vi "Turret_Execute.vi"() -> ()   [LabVIEW 2019]
uses:
  Globals/Turret_Globals.vi
  <vilib>/Rock Robotics/WPI/ThirdParty/REV Robotics/SPARK MAX/Typedef/Spark MAX Control Type.ctl
panel:
  out "Turret_Spin_Speed":dbl
  in  "turret_spin_encoder":dbl
  in  "t_x":dbl
  in  "Kp Aim":dbl=0.08
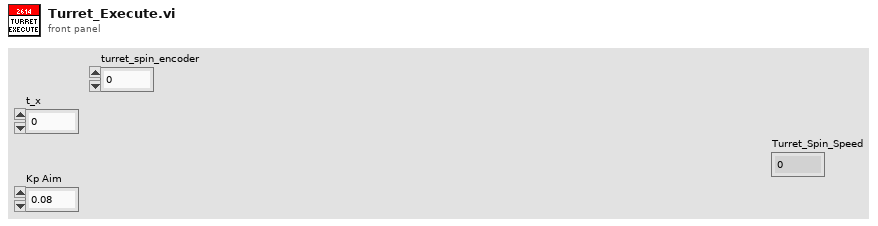
[diagram p1: front panel]
types:
  T1 = typedef "WPI_MotorControlDeviceRef.ctl" = cluster{"DeviceStatus":errorcluster, "Type":T2, "PWM":cluster{"PWM Channel":T3, "DeadBand":T4}, "CAN":cluster{"Device Number":u8, "SetOutput VI Ref":variant, "GetOutput VI Ref":variant, "Enable VI Ref":variant, "Disable VI Ref":variant, "Data":variant}, "Invert":bool, "DIO PWM":cluster{"PWM \"Enable\" Channel":T3, "DIOChannel":T5, "PWM Rate":dbl}}
  T2 = typedef "WPI_MotorControlType.ctl" = enum16{"PWM", "CAN", "DIO PWM"}
  T3 = typedef "FPGA_DIOPWMChannel.ctl" = enum8{"PWM 0", "PWM 1", "PWM 2", "PWM 3", "PWM 4", "PWM 5", "PWM 6", "PWM 7", "PWM 8", "PWM 9", "PWM MXP 0", "PWM MXP 1", "PWM MXP 2", "PWM MXP 3", "PWM MXP 4", "PWM MXP 5", "PWM MXP 6", "PWM MXP 7", "PWM MXP 8", "PWM MXP 9", "Invalid"}
  T4 = typedef "WPI_PWMDeadband.ctl" = cluster{"Name":string, "maxPositivePwm":i32, "minPositivePwm":i32, "centerPwm":i32, "maxNegativePwm":i32, "minNegativePwm":i32, "angularRange":u16}
  T5 = typedef "FPGA_DIOChannel.ctl" = enum8{"DIO 0", "DIO 1", "DIO 2", "DIO 3", "DIO 4", "DIO 5", "DIO 6", "DIO 7", "DIO 8", "DIO 9", "DIO MXP 0", "DIO MXP 1", "DIO MXP 2", "DIO MXP 3", "DIO MXP 4", "DIO MXP 5", "DIO MXP 6", "DIO MXP 7", "DIO MXP 8", "DIO MXP 9", "DIO MXP 10", "DIO MXP 11", "DIO MXP 12", "DIO MXP 13", "DIO MXP 14", "DIO MXP 15", "SPI Port CS1", "SPI Port CS2", "SPI Port CS3", "SPI Port MISO", "SPI Port MOSI", "Invalid"}
  T6 = typedef "Spark MAX Control Type.ctl" = enum16{"Percent VBus", "Voltage", "Velocity", "Position", "Smart Motion", "Current", "Smart Velocity"}
  T7 = typedef "Turret_Cluster.ctl" = cluster{"Auto-Target?":bool, "Control_State":T8, "Turret_Spin_Speed":dbl, "Turret_Spin_Speed_Control?":bool}
  T8 = typedef "Turret_States.ctl" = enum16{"Manual_Percent_Voltage", "Manual_Speed_Control", "Auto-Target"}
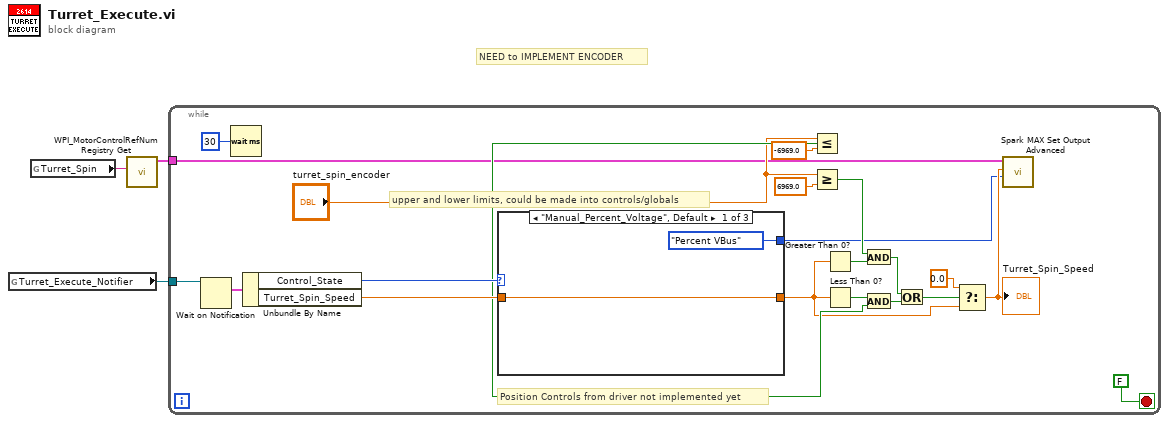
[diagram p0: block diagram]
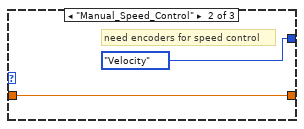
[diagram p2: hidden frame]
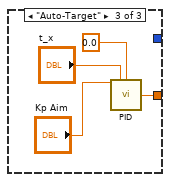
[diagram p3: hidden frame]
diagram:
  # "NEED to IMPLEMENT ENCODER"
  n1 = global read "Turret_Globals.vi" "Turret_Execute_Notifier"() -> (w3:refnum<notifier>)
  n2 = global read "Turret_Globals.vi" "Turret_Spin"() -> (w2:string)
  n3 = call <vilib>:"WPI_MotorControlRefNum Registry Get.vi"("refnum name"=w2) -> ("MotorControlDevRef"=w1:T1)  [unwired: 9 in, 1 out]
  n4 = while {
    tunnel: w3 -> [w23]
    tunnel: w1 -> [w6]
    stop <- FALSE stop-if-true
    # "Position Controls from driver not implemented yet"
    # "upper and lower limits, could be made into controls/globals"
    n5 = Wait on Notification(notifier=w23) -> (notification=w22:T7)  [unwired: 3 in, 3 out]
    n6 = Wait (ms)(milliseconds to wait=u32 30) -> ()  [unwired: 1 out]
    n7 = Unbundle By Name(w22) -> ("Control_State"=w21:T8, "Turret_Spin_Speed"=w20:dbl)
    n8 = case shown="\"Manual_Percent_Voltage\", Default" w21 {
      tunnel: w20 -> [w26 w27 _]
      tunnel: [w26 w27 w31] -> w11
      tunnel: [Spark_MAX_Control_Type."Percent VBus" ("Control Mode") Spark_MAX_Control_Type."Velocity" ("Control Mode") _] -> w4
      frame "Manual_Percent_Voltage", Default {
      }
      frame "Manual_Speed_Control" {
        # "need encoders for speed control"
      }
      frame "Auto-Target" {
        n9 = call "PID.vi"("Kp"="Kp Aim", "Process Variable"="t_x", "Goal"=0.0) -> ("Command"=w31:dbl)  [unwired: 10 in, 2 out]
      }
    }
    n10 = Less Or Equal?(x="turret_spin_encoder", y=-6969.0) -> (x <= y?=w17:bool)
    n11 = Greater Or Equal?(x="turret_spin_encoder", y=6969.0) -> (x >= y?=w19:bool)
    n12 = Greater Than 0?(x=w11) -> (x > 0?=w18:bool)
    n13 = Less Than 0?(x=w11) -> (x < 0?=w16:bool)
    n14 = And(x=w19, y=w18) -> (x .and. y?=w14:bool)
    n15 = And(x=w16, y=w17) -> (x .and. y?=w15:bool)
    n16 = Or(x=w14, y=w15) -> (x .or. y?=w13:bool)
    n17 = Select(t=0.0, s=w13, f=w11) -> (s? t:f=w5:dbl)
    "Turret_Spin_Speed" <- w5
    n18 = call <vilib>:"Spark MAX Set Output Advanced.vi"("Control Mode"=w4, "Setpoint"=w5, "MotorControlDevRef"=w6) -> ()  [unwired: 7 in, 2 out]
  }
